vi "Actor Core.vi"(8 "error in":errorcluster, 11 "Time Protocol":refnum<class "Time Protocol.lvclass">) -> (0 "error out":errorcluster, 3 "Actor out":refnum<class "Actor.lvclass">)   [LabVIEW 2013, in "Time Protocol Actor.lvlib" / "Time Protocol.lvclass"]
doc: "This is Actor Core.vi, the main message handling loop for Actors. An actor usually just sits in this loop and processes messages as they arrive. Any error returned by the message Do.vi call will stop the loop, with error code 43 as the canonical signal to stop with no error sent to caller. Descendants may override that in Handle Error.vi."
uses:
  Time Protocol.lvclass
  PluginInterface/Actor Framework.lvlibp/Actor/Actor.lvclass
  Time Protocol.lvclass/Time Protocol.ctl
  PluginInterface/PluginInterface.lvlibp/PluginInterfaceClass/PluginInterface.lvclass
  Write Code.vi
  Write History.vi
  Write Open.vi
  Write Path.vi
  Write State.vi
  PluginInterface/PluginInterface.lvlibp/PluginInterfaceClass/Write VI Refnum.vi
  PluginInterface/Actor Framework.lvlibp/Message Enqueuer/Enqueue.vi
  Time Protocol Messages/Open Protocol Msg/Open Protocol Msg.lvclass
  Time Protocol Messages/Change Status Msg/Change Status Msg.lvclass
  Time Protocol Messages/Run Protocol Msg/Run Protocol Msg.lvclass
  PluginInterface/Actor Framework.lvlibp/Stop Msg/Stop Msg.lvclass
panel:
  in  "stop signal":bool
  out "File Path Control":path
  in  "Radio Buttons":T1(radio)=enum."Media Stop Button"
  in  "Open Button":bool
  out "Code":i32(listbox)
  out "History":i32(listbox)=2
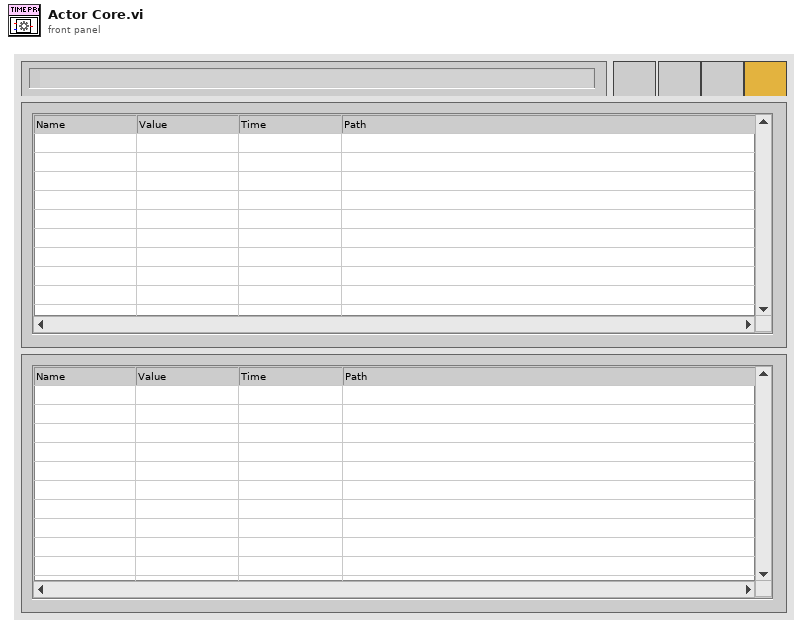
[diagram p1: front panel]
types:
  T1 = enum32{"Pause Button", "Play Button", "Media Stop Button"}
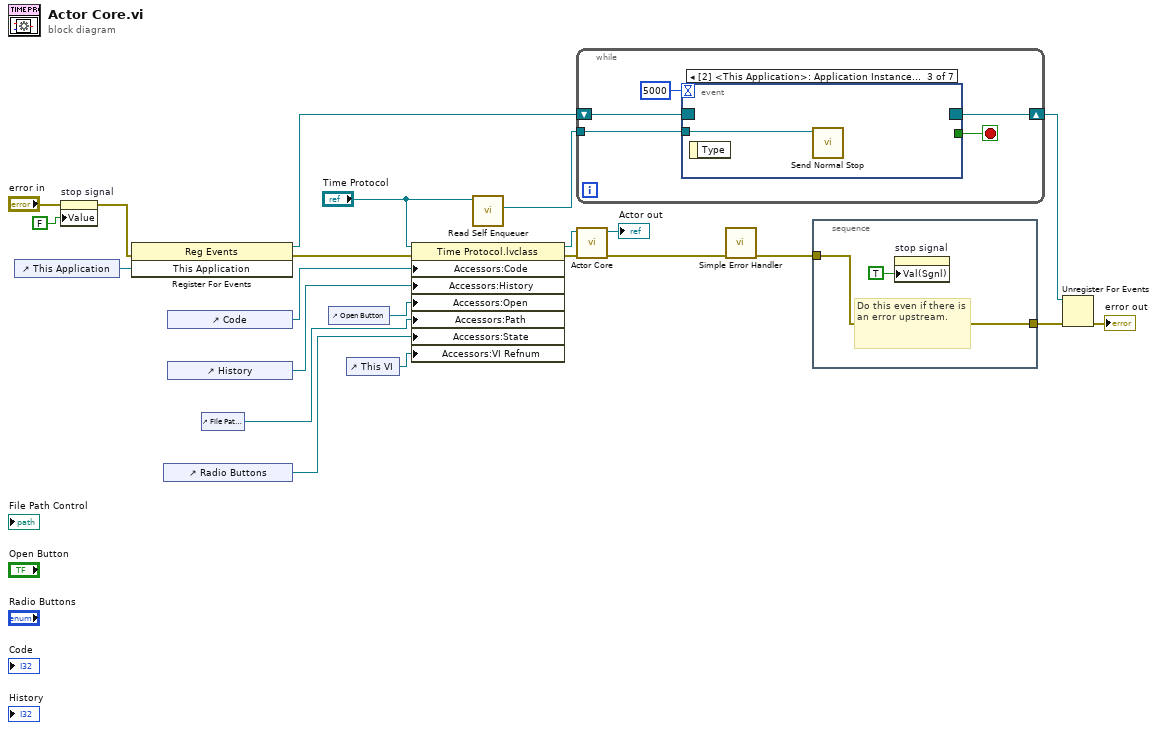
[diagram p0: block diagram]
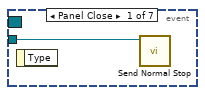
[diagram p2: hidden frame]
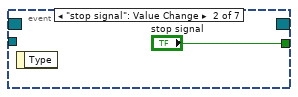
[diagram p3: hidden frame]
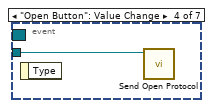
[diagram p4: hidden frame]
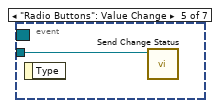
[diagram p5: hidden frame]
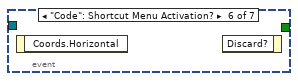
[diagram p6: hidden frame]
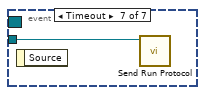
[diagram p7: hidden frame]
diagram:
  n1 = control-ref of="This Application"() -> (w15:refnum<vi>)
  n2 = property on="stop signal" class="Bool (strict)"(error in="error in", "Value"=FALSE ("stop")) -> (error out=w16:errorcluster)  [unwired: 1 in, 1 out]
  n3 = register-events(error in=w16, w15) -> (reference out=w19:refnum<event-registration>, error out=w1:errorcluster)  [unwired: 1 in]
  n4 = control-ref of="Radio Buttons"() -> (w6:refnum<vi>)
  n5 = control-ref of="Code"() -> (w2:refnum<vi>)
  n6 = control-ref of="History"() -> (w9:refnum<vi>)
  n7 = control-ref of="File Path Control"() -> (w7:refnum<vi>)
  n8 = control-ref of="Open Button"() -> (w8:refnum<vi>)
  n9 = control-ref of="This VI"() -> (w5:refnum<vi>)
  n10 = property class="Time Protocol.lvclass"(reference="Time Protocol", error in=w1, "Accessors:Code"=w2, "Accessors:History"=w9, "Accessors:Open"=w8, "Accessors:Path"=w7, "Accessors:State"=w6, "Accessors:VI Refnum"=w5) -> (reference out=w13:refnum<class "Time Protocol.lvclass">, error out=w14:errorcluster)
  n11 = call "Read Self Enqueuer.vi"("Actor"="Time Protocol") -> ("Self Enqueuer"=w3:refnum<class "Message Enqueuer.lvclass">)  [unwired: 10 in]
  n12 = while {
    tunnel: w3 -> [w27]
    shift-right: [w24] -> w18
    shift-left: w19 -> [w25]
    stop <- w26 stop-if-true
    n13 = event shown="[2] <This Application>: Application Instance Close" {
      selector: w25 -> [_ _ _ _ _ _ _]
      dyn-events: [_ _ _ _ _ _ _] -> w24
      timeout: 5000 -> [_ _ _ _ _ _ _]
      tunnel: w27 -> [w28 _ w30 w31 w32 _ w33]
      tunnel: [_ "stop signal" _ _ _ _ _] -> w26
      event Panel Close {
        n14 = event-data() -> ()  [unwired: 1 in, 1 out]
        n15 = call "Send Normal Stop.vi"("Message Enqueuer"=w28) -> ()  [unwired: 10 in, 1 out]
      }
      event "stop signal": Value Change {
        n16 = event-data() -> ()  [unwired: 1 in, 1 out]
      }
      event Application Instance Close {
        n17 = event-data() -> ()  [unwired: 1 in, 1 out]
        n18 = call "Send Normal Stop.vi"("Message Enqueuer"=w30) -> ()  [unwired: 10 in, 1 out]
      }
      event "Open Button": Value Change {
        n19 = event-data() -> ()  [unwired: 1 in, 1 out]
        n20 = call "Send Open Protocol.vi"("Message Enqueuer"=w31) -> ()  [unwired: 9 in, 2 out]
      }
      event "Radio Buttons": Value Change {
        n21 = event-data() -> ()  [unwired: 1 in, 1 out]
        n22 = call "Send Change Status.vi"("Message Enqueuer"=w32) -> ()  [unwired: 9 in, 2 out]
      }
      event "Code": Shortcut Menu Activation? {
        n23 = event-data() -> ()  [unwired: 1 in, 1 out]
        n24 = event-data() -> ()  [unwired: 2 in, 1 out]
      }
      event Timeout {
        n25 = event-data() -> ()  [unwired: 1 in, 1 out]
        n26 = call "Send Run Protocol.vi"("Message Enqueuer"=w33) -> ()  [unwired: 9 in, 2 out]
      }
    }
  }
  n27 = call-parent "Actor Core.vi"("error in"=w14, "Actor in"=w13) -> ("error out"=w21:errorcluster, "Actor out"=→"Actor out":refnum<class "Actor.lvclass">)  [unwired: 8 in]
  n28 = call <vilib>:"Simple Error Handler.vi"("error in (no error)"=w21) -> ("error out"=w20:errorcluster)  [unwired: 4 in, 4 out]
  n29 = stacked-sequence {
    tunnel: [w34] -> w17
    tunnel: w20 -> [w34]
    frame #0 {
      # "Do this even if there is an error upstream."
      n30 = property on="stop signal" class="Bool (strict)"("Val(Sgnl)"=TRUE ("stop")) -> ()  [unwired: 2 in, 2 out]
    }
  }
  n31 = Unregister For Events(event registration refnum=w18, error in=w17) -> (error out=→"error out":errorcluster)
